vi "Connect.vi"(10 "Grid in":refnum<class "Grid.lvclass">, 11 "Synapses in":refnum<class "Synapses.lvclass">) -> (2 "Grid out":refnum<class "Grid.lvclass">, 3 "Synapses  out":refnum<class "Synapses.lvclass">)   [LabVIEW 2013, in "Synapses.lvclass"]
doc: "This VI connects the neurons according to the synapses indicated. Returns the tables of pre and post neurons"
uses:
  Synapses.lvclass
  Cube/Grid.lvclass
  Synapses.lvclass/Synapses.ctl
  Cube/Grid.lvclass/Grid.ctl
  Neuron/Neuron.lvclass/Neuron.ctl
  Neuron/Get Neuron Properties.vi
  Utilities/id2coor.vi
panel:
  out "Progess":dbl
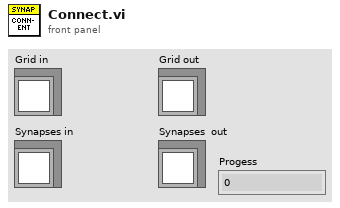
[diagram p1: front panel]
types:
  T1 = typedef "Synapses.ctl" = cluster{"Synapse":T2, "Pre_List":i32[][], "Post_List":i32[][], "Weight gain":dbl}
  T2 = typedef "Type of Synapses.ctl" = enum16{"MF to GC", "GO to GC", "GC to GO", "MF to GO", "GC to PC", "GC to BA", "PC to BA", "BA to PC", "BA to GO"}
  T3 = typedef "Type of Neuron.ctl" = enum16{"MF", "BA", "GO", "GC", "PC", "LU", "Glia (Dummy)"}
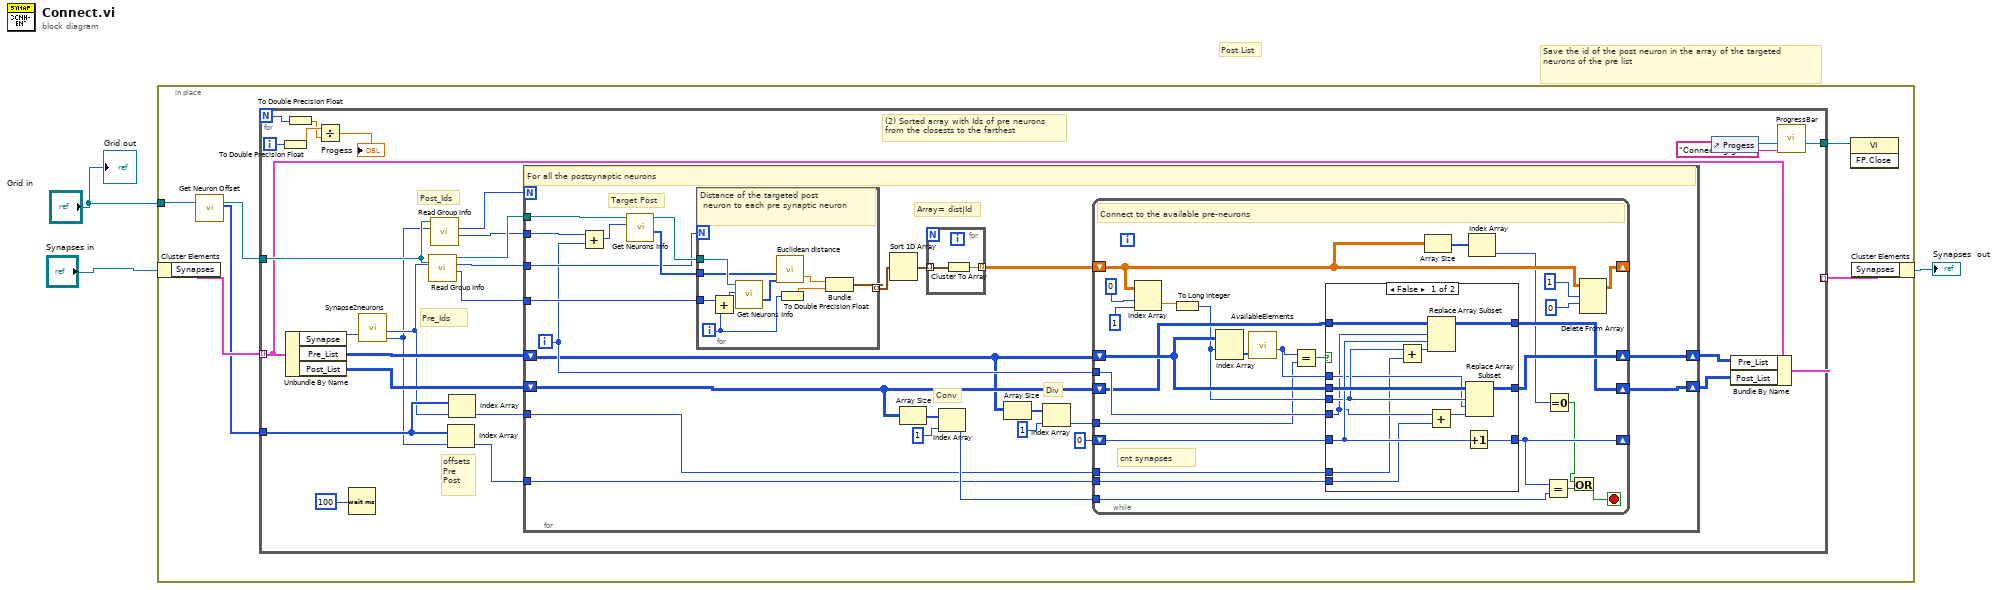
[diagram p0: block diagram]
diagram:
  # "Post List"
  # "Save the id of the post neuron in the array of the targeted neurons of the pre list"
  n1 = in-place {
    in-place-border: "Grid in" -> [w7]
    n2 = in-place-cluster #1("Synapses in") -> ("Synapses"=w9:T1[])
    n3 = call "Get Neuron Offset.vi"("Grid in"=w7) -> ("Neurons Offset Index"=w5:i32[], "Grid out"=w6:refnum<class "Grid.lvclass">)  [unwired: 9 in]
    n4 = for {
      N -> [w15]
      tunnel: w6 -> [w29]
      tunnel: w9 -> [w27] mode=indexing
      tunnel: [w24] -> w8 mode=indexing
      tunnel: w5 -> [w22]
      tunnel: [w11] -> w4
      i -> [w17]
      # "offsets\nPre\nPost"
      # "Post_Ids"
      # "Pre_Ids"
      # "(2) Sorted array with Ids of pre neurons\nfrom the closests to the farthest"
      n5 = To Double Precision Float(number=w17) -> (double precision float=w16:dbl)
      n6 = Unbundle By Name(w27) -> ("Synapse"=w33:T2, "Pre_List"=w30:i32[][], "Post_List"=w31:i32[][])
      n7 = To Double Precision Float(number=w15) -> (double precision float=w14:dbl)
      n8 = Divide(x=w16, y=w14) -> (x/y=→"Progess":dbl)
      n9 = Wait (ms)(milliseconds to wait=u32 100) -> ()  [unwired: 1 out]
      n10 = call "Synapse2neurons.vi"("Synapse"=w33) -> ("Post Neuron"=w20:T3, "Pre Neuron"=w21:T3)  [unwired: 4 in]
      n11 = call "Read Group Info.vi"("Neuron Type"=w21, "Grid in"=w29) -> ("Index"=w36:i32, "N"=w35:i32, "Grid out"=w34:refnum<class "Grid.lvclass">)  [unwired: 7 in]
      n12 = call "Read Group Info.vi"("Neuron Type"=w20, "Grid in"=w29) -> ("Index"=w32:i32, "N"=w28:i32)  [unwired: 7 in, 1 out]
      n13 = Index Array(array=w22, index=w20) -> (element=w18:i32)
      n14 = Index Array(array=w22, index=w21) -> (element=w19:i32)
      n15 = for {
        N: w28 -> [_]
        tunnel: w36 -> [w60]
        tunnel: w34 -> [w56]
        shift-right: [w52] -> w25
        shift-left: w30 -> [w40]
        shift-right: [w51] -> w26
        shift-left: w31 -> [w43]
        tunnel: w35 -> [w50]
        tunnel: w32 -> [w44]
        tunnel: w19 -> [w38]
        tunnel: w18 -> [w37]
        i -> [w48]
        # "Div"
        # "Conv"
        # "Array= dist|Id"
        # "Target Post"
        # "For all the postsynaptic neurons"
        n16 = Add(x=w44, y=w48) -> (x+y=w49:i32)
        n17 = call "Get Neurons Info.vi"("Neuron No"=w49, "Grid in"=w56) -> ("Position"=w59:i32[], "Grid out"=w55:refnum<class "Grid.lvclass">)  [unwired: 3 in, 5 out]
        n18 = for {
          N: w50 -> [_]
          tunnel: w60 -> [w109]
          tunnel: w55 -> [w114]
          tunnel: w59 -> [w107]
          tunnel: [w112] -> w58 mode=indexing
          i -> [w108]
          # "Distance of the targeted post\n neuron to each pre synaptic neuron"
          n19 = Add(x=w109, y=w108) -> (x+y=w110:i32)
          n20 = call "Get Neurons Info.vi"("Neuron No"=w110, "Grid in"=w114) -> ("Position"=w106:i32[])  [unwired: 3 in, 6 out]
          n21 = call "Euclidean distance.vi"("Position"=w107, "Position 2"=w106) -> ("Distance"=w113:dbl)  [unwired: 4 in]
          n22 = To Double Precision Float(number=w108) -> (double precision float=w111:dbl)
          n23 = Bundle("Distance"=w113, w111) -> (w112:cluster{"Distance":dbl, dbl})  [unwired: 1 in]
        }
        n24 = Sort 1D Array(array=w58) -> (sorted array=w57:cluster{"Distance":dbl, dbl}[])
        n25 = Array Size(array=w43) -> (size(s)=w47:i32[])
        n26 = for {
          tunnel: w57 -> [w104] mode=indexing
          tunnel: [w105] -> w54 mode=indexing
          n27 = Cluster To Array(cluster=w104) -> (array=w105:dbl[])
        }
        n28 = Index Array(array=w47, index=1 ("dimension size")) -> (element=w45:i32)
        n29 = Array Size(array=w40) -> (size(s)=w41:i32[])
        n30 = Index Array(array=w41, index=1 ("dimension size")) -> (element=w39:i32)
        n31 = while {
          shift-right: [w82] -> _
          shift-left: w54 -> [w71]
          shift-right: [w72] -> _
          shift-left: 0 -> [w75]
          shift-right: [w76] -> w52
          shift-left: w40 -> [w79]
          tunnel: w48 -> [w77]
          shift-right: [w73] -> w51
          shift-left: w43 -> [w74]
          tunnel: w45 -> [w64]
          tunnel: w39 -> [w63]
          tunnel: w38 -> [w62]
          tunnel: w37 -> [w61]
          stop <- w83 stop-if-true
          # "cnt synapses"
          # "Connect to the available pre-neurons"
          n32 = Index Array(array=w71, index (row)=0, index (col)=1 ("disabled index (col)")) -> (element=w78:dbl)
          n33 = To Long Integer(number=w78) -> (32bit integer=w67:i32)
          n34 = Index Array(array=w79, index (row)=w67) -> (element=w84:i32[])  [unwired: 1 in]
          n35 = call "AvailableElements.vi"("Array"=w84) -> ("No Available"=w65:i32)  [unwired: 3 in, 1 out]
          n36 = Equal?(x=w65, y=w63) -> (x = y?=w66:bool)
          n37 = case shown="False" w66 {
            tunnel: w79 -> [w100 w102]
            tunnel: w67 -> [w94 _]
            tunnel: w65 -> [w93 _]
            tunnel: w77 -> [w92 _]
            tunnel: [w99 w102] -> w76
            tunnel: w75 -> [w95 w103]
            tunnel: [w98 w103] -> w72
            tunnel: w74 -> [w97 w101]
            tunnel: [w96 w101] -> w73
            tunnel: w62 -> [w88 _]
            tunnel: w61 -> [w89 _]
            frame False {
              n38 = Add(x=w94, y=w88) -> (x+y=w90:i32)
              n39 = Replace Array Subset(array=w97, new element=w90, index (row)=w92, index (col)=w95) -> (w96:i32[][])
              n40 = Add(x=w92, y=w89) -> (x+y=w91:i32)
              n41 = Increment(x=w95) -> (x+1=w98:i32)
              n42 = Replace Array Subset(array=w100, new element=w91, index (row)=w94, index (col)=w93) -> (w99:i32[][])
            }
            frame True {
            }
          }
          n43 = Array Size(array=w71) -> (size(s)=w69:i32[])
          n44 = Index Array(array=w69) -> (element=w68:i32)  [unwired: 1 in]
          n45 = Equal?(x=w72, y=w64) -> (x = y?=w87:bool)
          n46 = Equal To 0?(x=w68) -> (x = 0?=w70:bool)
          n47 = Or(x=w70, y=w87) -> (x .or. y?=w83:bool)
          n48 = Delete From Array(array=w71, length=1, index (row)=0) -> (array with subset deleted=w82:dbl[][])  [unwired: 1 in, 1 out]
        }
      }
      n49 = control-ref of="Progess"() -> (w12:refnum<vi>)
      n50 = Bundle By Name(cluster=w27, "Pre_List"=w25, "Post_List"=w26) -> (w24:T1)
      n51 = call "ProgressBar.vi"("msgIn"="Connecting grid", "Progress"=w12) -> ("This VI"=w11:refnum<vi>)  [unwired: 9 in]
    }
    n52 = invoke class="VI" method="FP.Close"(reference=w4) -> ()  [unwired: 2 in, 3 out]
    n53 = in-place-cluster #1("Synapses"=w8) -> (→"Synapses  out":refnum<class "Synapses.lvclass">)
  }
  "Grid out" <- "Grid in"
